vi "LaunchGenerator.vi"   [LabVIEW 2021]
uses:
  Generator/Generator/Generator.lvclass
  C:/Program Files (x86)/National Instruments/LabVIEW 2021/vi.lib/ActorFramework/Actor/Actor.lvclass
  <vilib>/ActorFramework/Message Enqueuer/Message Enqueuer.lvclass/Message Enqueuer.ctl
  <vilib>/ActorFramework/Message Enqueuer/Enqueue.vi
  Generator/Generator Messages/GetRandomString Msg/GetRandomString Msg.lvclass
  C:/Program Files (x86)/National Instruments/LabVIEW 2021/vi.lib/ActorFramework/Message/Message.lvclass
  Generator/Generator Messages/GetRandomNum Msg/GetRandomNum Msg.lvclass
  Generator/Generator Messages/GetDateTimeString Msg/GetDateTimeString Msg.lvclass
  <vilib>/ActorFramework/Stop Msg/Stop Msg.lvclass
  <vilib>/ActorFramework/Message Priority Queue/Priority Enqueue.vi
  <vilib>/ActorFramework/Actor/Actor.lvclass
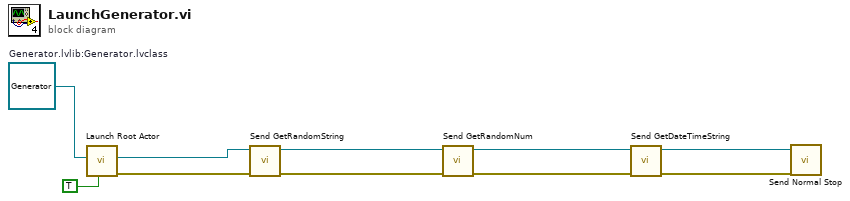
[diagram p0: block diagram]
diagram:
  w10 = refnum<class "Generator.lvclass"> refnum  # Generator.lvlib:Generator.lvclass
  n1 = call <vilib>:"Launch Root Actor.vi"("Open Actor Core front panel? (F)"=TRUE, "Actor"=w10) -> ("error out"=w8:errorcluster, "Actor's Enqueuer"=w9:refnum<class "Message Enqueuer.lvclass">)  [unwired: 8 in]
  n2 = call "Send GetRandomString.vi"("error in (no error)"=w8, "Message Enqueuer"=w9) -> ("error out"=w6:errorcluster, "Message Enqueuer out"=w7:refnum<class "Message Enqueuer.lvclass">)  [unwired: 8 in]
  n3 = call "Send GetRandomNum.vi"("error in (no error)"=w6, "Message Enqueuer"=w7) -> ("error out"=w4:errorcluster, "Message Enqueuer out"=w5:refnum<class "Message Enqueuer.lvclass">)  [unwired: 8 in]
  n4 = call "Send GetDateTimeString.vi"("error in (no error)"=w4, "Message Enqueuer"=w5) -> ("error out"=w1:errorcluster, "Message Enqueuer out"=w2:refnum<class "Message Enqueuer.lvclass">)  [unwired: 8 in]
  n5 = call <vilib>:"Send Normal Stop.vi"("error in (no error)"=w1, "Message Enqueuer"=w2) -> ()  [unwired: 9 in, 1 out]
